vi "Main Tclk.vi"() -> ()   [LabVIEW 2018] (continued)
                n3941 = case shown="True" w3026 {
                  tunnel: w3025 -> [w3034 w3039]
                  tunnel: [w3034 w3039] -> w3024
                  frame False {
                  }
                  frame True {
                    n3942 = Two Button Dialog(message="Are you sure to resume from the last recipe and milling position?") -> (T button?=w3035:bool)  [unwired: 2 in]
                    n3943 = local read "Milling para"() -> (w3036:T35)
                    n3944 = Bundle By Name(cluster=w3036, "Mill start from Last"=w3035) -> (w3037:T35)
                    n3945 = local write "Milling para"(w3037) -> ()
                  }
                }
                n3946 = case shown="2" w3021 {
                  frame 0, Default {
                  }
                  frame 2 {
                    n3947 = local read "Api"() -> (w3033:refnum<k7>)
                    n3948 = local read "FIB Milling Probe"() -> (w3031:string)
                    n3949 = call "SmartSEM Remote API set string.vi"("vValue"=w3031, "lpszParam"="DP_FIB_IMAGE_PROBE", "Api"=w3033) -> ("Api out"=w3030:refnum<k7>)  [unwired: 7 in, 1 out]
                    n3950 = call "SmartSEM Remote API set float.vi"("vValue"="FIB Milling Objective (V)", "lpszParam"="AP_FIB_OBJECTIVE_POTENTIAL", "Api"=w3030) -> ()  [unwired: 7 in, 2 out]
                  }
                }
                n3951 = local write "3D FIB-SEM"(w3024) -> ()
                n3952 = local write "FIB"(w3024) -> ()
                n3953 = case shown="True" w3024 {
                  frame False {
                  }
                  frame True {
                    n3954 = local read "Email Alert Recipients"() -> (w3051:string[])
                    n3955 = local read "Email recipents file"() -> (w3048:path)
                    n3956 = local read "Post #1up"() -> (w3045:tag)
                    n3957 = local read "Post #1down"() -> (w3043:tag)
                    n3958 = local read "Post #2up"() -> (w3044:tag)
                    n3959 = local read "Post #2down"() -> (w3042:tag)
                    n3960 = local write "FIB slice #"(u32 0 ("slice #")) -> ()
                    n3961 = local write "Start FIB HV DataLog"(TRUE ("Start FIB HV DataLog")) -> ()
                    n3962 = local write "Status Tabs"(T11."Status" ("Status Tabs")) -> ()
                    n3963 = Open/Create/Replace File(file path (use dialog)=w3048, operation (0:open)=T49."replace or create") -> (refnum out=w3049:refnum<file>, error out=w3050:errorcluster)  [unwired: 4 in, 1 out]
                    n3964 = call "SEM shutter.vi"("Shutter close"=TRUE, "Shutter AO4"=w3042, "Shutter AO3"=w3044, "Shutter AO2"=w3043, "Shutter AO1"=w3045) -> ()  [unwired: 6 in, 1 out]
                    n3965 = Write to Text File(file (use dialog)=w3049, text=w3051, error in=w3050) -> (refnum out=w3052:refnum<file>, error out=w3053:errorcluster)  [unwired: 1 in, 1 out]
                    n3966 = Close File(refnum=w3052, error in=w3053) -> ()  [unwired: 2 out]
                  }
                }
              }
            }
          }
          event "Pause for reheat": Value Change {
            n3967 = event-data() -> ("NewVal"=w3055:bool)  [unwired: 6 out]
            n3968 = case shown="False" w3055 {
              frame False {
                w3058 = u8 0 ("FI below limit counts")
                n3969 = local read "Machine Type"() -> (w3056:u8)
                n3970 = case shown="1" w3056 {
                  tunnel: [w3064 w3072 w3073] -> w3057
                  frame 0, Default {
                    n3971 = for {
                      N: 10 -> [_]
                      tunnel: [w3069] -> w3066 mode=indexing
                      n3972 = shared-variable ".\\Zeiss Library.lvlib\\Logs"() -> (w3071:sgl[])  [unwired: 1 in, 1 out]
                      n3973 = Wait Until Next ms Multiple(millisecond multiple=u32 10) -> ()  [unwired: 1 out]
                      n3974 = Index Array(array=w3071, index=0) -> (element=w3069:sgl)
                    }
                    n3975 = call-poly <vilib>:"Basic Averaged DC-RMS.vi"("signal in"=w3066) -> ("DC value"=w3065:dbl)  [unwired: 7 in, 3 out]
                    n3976 = To Single Precision Float(number=w3065) -> (single precision float=w3064:sgl)
                  }
                  frame 1 {
                    n3977 = local read "Faraday Cup (nA)"() -> (w3072:sgl)
                  }
                  frame 2 {
                    n3978 = for {
                      N: 10 -> [_]
                      tunnel: [w3078] -> w3075 mode=indexing
                      n3979 = shared-variable ".\\Zeiss Library.lvlib\\Logs"() -> (w3080:sgl[])  [unwired: 1 in, 1 out]
                      n3980 = Wait Until Next ms Multiple(millisecond multiple=u32 10) -> ()  [unwired: 1 out]
                      n3981 = Index Array(array=w3080, index=0) -> (element=w3078:sgl)
                    }
                    n3982 = call-poly <vilib>:"Basic Averaged DC-RMS.vi"("signal in"=w3075) -> ("DC value"=w3074:dbl)  [unwired: 7 in, 3 out]
                    n3983 = To Single Precision Float(number=w3074) -> (single precision float=w3073:sgl)
                  }
                }
                n3984 = local write "FI below limit counts"(w3058) -> ()
                n3985 = local write "FIB CL I out of bound counts"(w3058) -> ()
                n3986 = shared-variable ".\\Zeiss Library.lvlib\\Faraday Cup before mill"(w3057) -> ()  [unwired: 1 in, 1 out]
                n3987 = local write "Faraday Cup before mill"(w3057) -> ()
                n3988 = call <vilib>:"Three Button Dialog.vi"("Allow user to close window? (TRUE)"=FALSE, "Center Button Text (\"No\")"="Manual Re-engage" ("T button name (\"OK\")"), "Left Button Text (\"Yes\")"="Auto Re-engage" ("T button name (\"OK\")"), "message"="Reheat finish and ready to re-engage?") -> ("Which Button?"=w3060:T78)  [unwired: 7 in]
                n3989 = case shown="\"Left Button\"" w3060 {
                  frame "Left Button" {
                    n3990 = stacked-sequence {
                      frame #0 {
                        w3093 = dbl[] [] ("Re-engage Delta X array")
                        w3082 = u8 0 ("Re-engage X shift")
                        w3085 = TRUE ("Auto re-engage")
                        n3991 = local read "X shift from last"() -> (w3087:dbl)
                        n3992 = local read "Y shift from last"() -> (w3091:dbl)
                        n3993 = local read "Reheat from last"() -> (w3088:bool)
                        n3994 = local read "FIB-SEM Angle"() -> (w3096:dbl)
                        n3995 = Get Date/Time In Seconds() -> (seconds since 1Jan1904=w3094:timestamp)
                        "Re-engage time" <- w3094
                        n3996 = local read "Pre-reheat time"() -> (w3097:timestamp)
                        n3997 = Subtract(x=w3094, y=w3097) -> (x-y=w3098:dbl)
                        n3998 = expression code="x/60"(w3098) -> (w3099:dbl)
                        n3999 = expression code="cos(x*pi/180)"(w3096) -> (w3095:dbl)
                        n4000 = Select(t=w3087, s=w3088, f=0.0 ("Re-engage X shift")) -> (s? t:f=w3090:dbl)
                        n4001 = shared-variable ".\\Zeiss Library.lvlib\\FIB PID reset"(w3085) -> ()  [unwired: 1 in, 1 out]
                        n4002 = Natural Logarithm(1:w3099) -> (0:w3101:dbl)
                        n4003 = local write "Re-engage X shift (um)"(w3090) -> ()
                        n4004 = local write "Status message"("Auto re-engaging ..." ("Status message")) -> ()
                        n4005 = Compound Arithmetic op=MULTIPLY(w3095, w3101, 2.5 ("value"), 0.0 ("value")) -> (w3092:dbl)
                        n4006 = Select(t=w3091, s=w3088, f=w3092) -> (s? t:f=w3086:dbl)
                        n4007 = local write "Re-engage Y shift (um)"(w3086) -> ()
                        n4008 = local write "Status Tabs"(T11."Status" ("Status Tabs")) -> ()
                        n4009 = local write "Re-engage counts"(w3082) -> ()
                        n4010 = local write "Recovered counts"(w3082) -> ()
                        n4011 = local write "Last re-engage count"(w3082) -> ()
                        "Auto re-engage" <- w3085
                        "Re-engage Delta X array" <- w3093
                        "Re-engage Delta Y array" <- w3093
                        "Re-engage Y shift array" <- w3093
                        "Re-engage X shift array" <- w3093
                      }
                      frame #1 {
                        w3105 = TRUE ("Reset WD")
                        w3106 = FALSE ("Reheat")
                        n4012 = local write "Config Tabs"(T24."SEM" ("Config Tabs")) -> ()
                        n4013 = local write "Image Tabs"(T37."Detector A" ("Image Tabs")) -> ()
                        n4014 = local write "Pause for reheat"(w3106) -> ()
                        n4015 = local write "Mill Manual Pause"(w3106) -> ()
                        n4016 = local write "Reheat from last"(w3106) -> ()
                        n4017 = property on="Mill Manual Pause" class="Bool (strict)"("DisabledEnum"=T44."Enabled" ("Disabled")) -> ()  [unwired: 2 in, 2 out]
                        n4018 = local write "3D image paused armed"(w3105) -> ()
                        n4019 = local write "SW error warning armed"(w3105) -> ()
                        n4020 = local write "Temperature warning armed"(w3105) -> ()
                        n4021 = local read "Alert Settings"() -> (→"Prior Alert Settings":T36)
                      }
                    }
                  }
                  frame "Center Button", Default {
                    w3111 = TRUE ("Reset WD")
                    w3113 = FALSE ("Reheat")
                    n4022 = local write "3D image paused armed"(w3111) -> ()
                    n4023 = local write "Reset Focus"(w3111) -> ()
                    n4024 = local write "SW error warning armed"(w3111) -> ()
                    n4025 = shared-variable ".\\Zeiss Library.lvlib\\FIB PID reset"(w3111) -> ()  [unwired: 1 in, 1 out]
                    n4026 = local write "Temperature warning armed"(w3111) -> ()
                    n4027 = local write "Config Tabs"(T24."SEM" ("Config Tabs")) -> ()
                    n4028 = local write "Status Tabs"(T11."Status" ("Status Tabs")) -> ()
                    n4029 = local write "Image Tabs"(T37."Detector A" ("Image Tabs")) -> ()
                    n4030 = local write "Pause for reheat"(w3113) -> ()
                    n4031 = local write "Mill Manual Pause"(w3113) -> ()
                    n4032 = local write "Reheat from last"(w3113) -> ()
                    n4033 = property on="Mill Manual Pause" class="Bool (strict)"("DisabledEnum"=T44."Enabled" ("Disabled")) -> ()  [unwired: 2 in, 2 out]
                    n4034 = local write "Status message"("Manual re-engaging ..." ("Status message")) -> ()
                  }
                  frame "Right Button" {
                    n4035 = local write "Pause for reheat"(TRUE ("Reheat request")) -> ()
                  }
                }
              }
              frame True {
                n4036 = local read "Mill Manual Pause"() -> (w3129:bool)
                n4037 = Get Date/Time In Seconds() -> (seconds since 1Jan1904=w3127:timestamp)
                n4038 = local read "3D FIB-SEM Files"() -> (w3119:path)
                n4039 = local read "Re-engage Files"() -> (w3117:path)
                n4040 = local read "Last good FI"() -> (w3126:sgl)
                n4041 = case shown="False" w3129 {
                  frame False {
                    n4042 = stacked-sequence {
                      frame #0 {
                        n4043 = local write "Pause for reheat"(FALSE ("Reheat")) -> ()
                      }
                      frame #1 {
                        n4044 = Two Button Dialog(message="Pause to reheat FIB source?") -> (T button?=w3131:bool)  [unwired: 2 in]
                        n4045 = local write "Pause for reheat"(w3131) -> ()
                        n4046 = case shown="True" w3131 {
                          frame False {
                          }
                          frame True {
                            n4047 = local write "Reheat completed"(FALSE ("Reheat completed")) -> ()
                            n4048 = local write "Status message"("Pausing for FIB reheat ..." ("Status message")) -> ()
                            n4049 = property on="Pause for reheat" class="Bool (strict)"("DisabledEnum"=T44."Disabled and Grayed Out" ("Disabled")) -> ()  [unwired: 2 in, 2 out]
                          }
                        }
                      }
                    }
                  }
                  frame True {
                    n4050 = property on="Mill Manual Pause" class="Bool (strict)"("DisabledEnum"=T44."Disabled and Grayed Out" ("Disabled")) -> ()  [unwired: 2 in, 2 out]
                  }
                }
                n4051 = local read "SEM Scan Parameters"() -> (w3128:T26)
                n4052 = Build Path(base path=w3119, name or relative path="LG low res.png") -> (appended path=w3120:path)
                n4053 = Build Path(base path=w3117, name or relative path="pre.png") -> (appended path=w3121:path)
                n4054 = local write "Pre-reheat time"(w3127) -> ()
                n4055 = Copy(9:TRUE ("overwrite (F)"), 10:w3121, 11:w3120) -> ()  [unwired: 2 in, 3 out]
                n4056 = local write "Pre-reheat FI"(w3126) -> ()
                n4057 = Unbundle By Name(w3128) -> ("X center (um)"=w3125:sgl, "Y center (um)"=w3124:sgl, "Y stig"=w3123:sgl[][])
                n4058 = local write "Pre-reheat X center (um)"(w3125) -> ()
                n4059 = local write "Pre-reheat Y center (um)"(w3124) -> ()
                n4060 = local write "Pre-reheat Y stig"(w3123) -> ()
              }
            }
          }
          event "FIB Imaging": Mouse Down {
            n4061 = event-data() -> ("PlatMods"=w3138:T77)  [unwired: 7 out]
            n4062 = Unbundle By Name(w3138) -> ("Shift"=→"FIB single scan":bool)
          }
          event "FIB Imaging": Value Change {
            n4063 = event-data() -> ("NewVal"=w3139:bool)  [unwired: 5 out]
            n4064 = case shown="True" w3139 {
              selector: w3139 -> [w3140 _]
              frame False {
                n4065 = local write "Unfreeze"(w3140) -> ()
                n4066 = stacked-sequence {
                  frame #0 {
                    n4067 = shared-variable "My Computer\\Zeiss Library.lvlib\\Realtime Imaging stop"(TRUE ("Realtime Imaging stop")) -> ()  [unwired: 1 in, 1 out]
                  }
                  frame #1 {
                    n4068 = disable-structure shown="Disabled" {
                      frame Disabled {
                        n4069 = local read "Machine Type"() -> (w3142:u8)
                        n4070 = case shown="1" w3142 {
                          frame 0, Default {
                          }
                          frame 1 {
                            n4071 = stacked-sequence {
                              frame #0 {
                                n4072 = Wait (ms)(milliseconds to wait=u32 1000) -> ()  [unwired: 1 out]
                              }
                              frame #1 {
                                w3144 = TRUE ("Initialization")
                                n4073 = local read "COM port"() -> (w3150:refnum<visa-resource-name>)
                                n4074 = call "FIB mode.vi"("Initialization"=w3144, "FIB mode"=T10."SEM", "COM port in"=w3150) -> ("COM port out"=w3149:refnum<visa-resource-name>)  [unwired: 7 in, 1 out]
                                n4075 = call "Remcon32 command.vi"("SEM command"="edx 0", "COM port in"=w3149) -> ("COM port out"=w3148:refnum<visa-resource-name>)  [unwired: 6 in, 3 out]
                                n4076 = call "Remcon32 command.vi"("Close session"=w3144, "SEM command"="frez", "COM port in"=w3148) -> ()  [unwired: 5 in, 4 out]
                              }
                            }
                          }
                          frame 2 {
                          }
                        }
                      }
                      frame Enabled {
                      }
                    }
                  }
                  frame #2 {
                    w3152 = T44."Enabled" ("Disabled")
                    n4077 = local write "Status message"("standby" ("Status message")) -> ()
                    n4078 = property on="Pre image" class="Bool (strict)"("DisabledEnum"=w3152) -> ()  [unwired: 2 in, 2 out]
                    n4079 = property on="Post image" class="Bool (strict)"("DisabledEnum"=w3152) -> ()  [unwired: 2 in, 2 out]
                    n4080 = local read "FIB"() -> (w3153:bool)
                    n4081 = property on="Mill Manual Pause" class="Bool (strict)"("DisabledEnum"=w3152) -> ()  [unwired: 2 in, 2 out]
                    n4082 = case shown="False" w3153 {
                      tunnel: w3152 -> [w3154 _]
                      frame False {
                        n4083 = property on="Mill" class="Bool (strict)"("DisabledEnum"=w3154) -> ()  [unwired: 2 in, 2 out]
                      }
                      frame True {
                      }
                    }
                  }
                }
              }
              frame True {
                n4084 = local read "Machine Type"() -> (w3156:u8)
                n4085 = case shown="2" w3156 {
                  tunnel: [TRUE ("true") w3168] -> w3155
                  frame 0, Default {
                  }
                  frame 2 {
                    n4086 = local read "Api"() -> (w3166:refnum<k7>)
                    n4087 = Two Button Dialog(message="Verify if FIB probe is at 50 pA") -> (T button?=w3168:bool)  [unwired: 2 in]
                    n4088 = call "SmartSEM Remote API set string.vi"("vValue"="FIB Imaging Probe", "lpszParam"="DP_FIB_IMAGE_PROBE", "Api"=w3166) -> ()  [unwired: 7 in, 2 out]
                  }
                }
                "Unfreeze" <- w3155
                n4089 = case shown="True" w3155 {
                  frame False {
                  }
                  frame True {
                    n4090 = stacked-sequence {
                      frame #0 {
                        n4091 = local read "Spot"() -> (w3157:bool)
                        n4092 = case shown="True" w3157 {
                          frame False {
                          }
                          frame True {
                            n4093 = local write "Spot"(FALSE ("Spot")) -> ()
                            n4094 = Wait (ms)(milliseconds to wait=u32 200) -> ()  [unwired: 1 out]
                          }
                        }
                      }
                      frame #1 {
                        w3162 = T44."Disabled and Grayed Out" ("Disabled")
                        n4095 = local write "Status message"("FIB Imaging" ("Status message")) -> ()
                        n4096 = local write "Image Tabs"(T37."FIB" ("Image Tabs")) -> ()
                        n4097 = local write "Status Tabs"(T11."FIB" ("Status Tabs")) -> ()
                        n4098 = property on="Pre image" class="Bool (strict)"("DisabledEnum"=w3162) -> ()  [unwired: 2 in, 2 out]
                        n4099 = property on="Post image" class="Bool (strict)"("DisabledEnum"=w3162) -> ()  [unwired: 2 in, 2 out]
                        n4100 = property on="Mill" class="Bool (strict)"("DisabledEnum"=w3162) -> ()  [unwired: 2 in, 2 out]
                        n4101 = property on="Mill Manual Pause" class="Bool (strict)"("DisabledEnum"=w3162) -> ()  [unwired: 2 in, 2 out]
                      }
                    }
                  }
                }
                n4102 = local write "FIB Imaging"(w3155) -> ()
              }
            }
          }
          event "Update": Value Change {
            n4103 = event-data() -> ("NewVal"=w3170:bool)  [unwired: 5 out]
            n4104 = case shown="True" w3170 {
              frame False {
              }
              frame True {
                n4105 = stacked-sequence {
                  frame #0 {
                    n4106 = local write "Unfreeze"(FALSE ("FIB beam blank")) -> ()
                    n4107 = shared-variable "My Computer\\Zeiss Library.lvlib\\Realtime Imaging stop"(TRUE ("Realtime Imaging stop")) -> ()  [unwired: 1 in, 1 out]
                  }
                  frame #1 {
                    n4108 = Wait (ms)(milliseconds to wait=u32 1000) -> ()  [unwired: 1 out]
                  }
                  frame #2 {
                    n4109 = local write "Unfreeze"(TRUE ("Realtime Imaging stop")) -> ()
                  }
                }
              }
            }
          }
          event "Reset": Value Change {
            n4110 = event-data() -> ("NewVal"=w3175:bool)  [unwired: 5 out]
            n4111 = case shown="True" w3175 {
              frame False {
              }
              frame True {
                n4112 = stacked-sequence {
                  frame #0 {
                    n4113 = local read "SEM HW Config"() -> (w3186:T9)
                    n4114 = local read "FIB HW Config"() -> (w3178:T23)
                    n4115 = Unbundle By Name(w3186) -> ("SEM X coil"=w3185:refnum<k15>)
                    n4116 = Unbundle By Name(w3178) -> ("FIB X coil"=w3177:tag)
                    n4117 = Type Cast(x=w3185) -> (*(type *) &x=w3184:string)  [unwired: 1 in]
                    n4118 = Type Cast(x=w3177) -> (*(type *) &x=w3179:string)  [unwired: 1 in]
                    n4119 = Match Pattern(string=w3184, regular expression="/") -> (before substring=w3182:string)  [unwired: 1 in, 3 out]
                    n4120 = Match Pattern(string=w3179, regular expression="/") -> (before substring=w3181:string)  [unwired: 1 in, 3 out]
                    n4121 = call <vilib>:"DAQmx Reset Device.vi"("device in"=w3182) -> ()  [unwired: 14 in, 1 out]
                    n4122 = call <vilib>:"DAQmx Reset Device.vi"("device in"=w3181) -> ()  [unwired: 14 in, 1 out]
                    n4123 = shared-variable ".\\Zeiss Library.lvlib\\Force tclk init"(TRUE ("Force tclk init")) -> ()  [unwired: 1 in, 1 out]
                  }
                  frame #1 {
                    n4124 = local read "FIB HW Config"() -> (w3194:T23)
                    n4125 = Unbundle By Name(w3194) -> ("Beam blank"=w3195:tag)
                    n4126 = local read "Api"() -> (w3187:refnum<k7>)
                    n4127 = call "FIB beam blank.vi"("Api"=w3187, "Beam blanked"=TRUE ("Ext on"), "lines"=w3195) -> ()  [unwired: 2 in, 1 out]
                    n4128 = local read "Post #1up"() -> (w3191:tag)
                    n4129 = local read "Post #1down"() -> (w3190:tag)
                    n4130 = local read "Post #2up"() -> (w3189:tag)
                    n4131 = local read "Post #2down"() -> (w3188:tag)
                    n4132 = call "SEM shutter.vi"("Shutter close"=FALSE, "Shutter AO4"=w3188, "Shutter AO3"=w3189, "Shutter AO2"=w3190, "Shutter AO1"=w3191) -> ()  [unwired: 6 in, 1 out]
                  }
                  frame #2 {
                    n4133 = local read "SEM HW Config"() -> (w3200:T9)
                    n4134 = Unbundle By Name(w3200) -> ("Detector FIB-NI auto switch"=w3201:tag)
                    n4135 = call-poly <vilib>:"DAQmx Create Virtual Channel.vi"("lines"=w3201) -> ("task out"=w3198:refnum<k21>, "error out"=w3199:errorcluster)  [unwired: 4 in, 9 out]
                    n4136 = call-poly <vilib>:"DAQmx Write.vi"("task/channels in"=w3198, "data"=FALSE, "error in"=w3199) -> ("task out"=w3196:refnum<k21>, "error out"=w3197:errorcluster)  [unwired: 1 in, 10 out]
                    n4137 = call <vilib>:"DAQmx Clear Task.vi"("task in"=w3196, "error in"=w3197) -> ()  [unwired: 14 out]
                  }
                  frame #3 {
                    n4138 = local read "FIB HW Config"() -> (w3205:T23)
                    n4139 = Unbundle By Name(w3205) -> ("FIB Ext Scan"=w3204:tag)
                    n4140 = call "FIB ext scan.vi"("Ext on"=FALSE, "FIB Ext Scan"=w3204) -> ()  [unwired: 9 in, 1 out]
                  }
                  frame #4 {
                    n4141 = local read "Machine Type"() -> (w3206:u8)
                    n4142 = case shown="2" w3206 {
                      frame 0, Default {
                      }
                      frame 1 {
                        w3207 = TRUE ("Initialization")
                        n4143 = local read "COM port"() -> (w3213:refnum<visa-resource-name>)
                        n4144 = call "FIB mode.vi"("Initialization"=w3207, "FIB mode"=T10."SEM", "COM port in"=w3213) -> ("COM port out"=w3212:refnum<visa-resource-name>)  [unwired: 7 in, 1 out]
                        n4145 = call "Remcon32 command.vi"("SEM command"="edx 0", "COM port in"=w3212) -> ("COM port out"=w3211:refnum<visa-resource-name>)  [unwired: 6 in, 3 out]
                        n4146 = call "Remcon32 command.vi"("Close session"=w3207, "SEM command"="frez", "COM port in"=w3211) -> ()  [unwired: 5 in, 4 out]
                      }
                      frame 2 {
                        n4147 = local read "Api"() -> (w3214:refnum<k7>)
                        n4148 = call "SmartSEM Remote API set float.vi"("vValue"=sgl 0.0, "lpszParam"="DP_PANEL_DISABLE", "Api"=w3214) -> ("Api out"=w3215:refnum<k7>)  [unwired: 7 in, 1 out]
                        n4149 = call "SmartSEM Remote API set float.vi"("vValue"=sgl 0.0, "lpszParam"="DP_JOYSTICK_DISABLE", "Api"=w3215) -> ()  [unwired: 7 in, 2 out]
                      }
                    }
                  }
                  frame #5 {
                    n4150 = local write "Reset"(FALSE ("Reset")) -> ()
                  }
                }
              }
            }
          }
          event "Off": Value Change {
            n4151 = event-data() -> ("NewVal"=w3221:bool)  [unwired: 6 out]
            n4152 = case shown="False" w3221 {
              tunnel: [FALSE ("T button?") w3224] -> w3222
              frame False {
              }
              frame True {
                n4153 = local read "FIB"() -> (w3225:bool)
                n4154 = Two Button Dialog(message="Stop Program?") -> (T button?=w3226:bool)  [unwired: 2 in]
                n4155 = case shown="True" w3225 {
                  tunnel: w3226 -> [w3228 w3229]
                  tunnel: [w3228 w3229] -> w3224
                  frame False {
                    n4156 = shared-variable "My Computer\\Zeiss Library.lvlib\\Stop"(w3228) -> ()  [unwired: 1 in, 1 out]
                    n4157 = shared-variable "My Computer\\Zeiss Library.lvlib\\Milling Stop"(w3228) -> ()  [unwired: 1 in, 1 out]
                    n4158 = shared-variable "My Computer\\Zeiss Library.lvlib\\Realtime Imaging stop"(w3228) -> ()  [unwired: 1 in, 1 out]
                    n4159 = local write "Stop"(w3228) -> ()
                    n4160 = local write "Off"(w3228) -> ()
                  }
                  frame True {
                    n4161 = shared-variable "My Computer\\Zeiss Library.lvlib\\Stop"(w3229) -> ()  [unwired: 1 in, 1 out]
                    n4162 = shared-variable "My Computer\\Zeiss Library.lvlib\\Milling Stop"(w3229) -> ()  [unwired: 1 in, 1 out]
                    n4163 = shared-variable "My Computer\\Zeiss Library.lvlib\\Realtime Imaging stop"(w3229) -> ()  [unwired: 1 in, 1 out]
                    n4164 = local write "Stop"(w3229) -> ()
                    n4165 = local write "Off"(w3229) -> ()
                  }
                }
              }
            }
          }
          event "SEM Scan Parameters": Value Change {
            w3231 = sgl[] [] ("Delta X array for stop limit")
            n4166 = event-data() -> ()  [unwired: 6 out]
            n4167 = local write "SW error warning armed"(FALSE ("SW error warning armed")) -> ()
            n4168 = local write "Cycle time array"(u32[] [] ("Cycle time array")) -> ()
            n4169 = local write "Cycle time est offset array"(i16[] [] ("Cycle time array")) -> ()
            n4170 = local write "Continued fine milling frames"(0 ("Continued fine milling frames")) -> ()
            n4171 = local write "FI array for stop limit"(w3231) -> ()
            n4172 = local write "Delta X array for stop limit"(w3231) -> ()
            n4173 = local write "Delta Y array for stop limit"(w3231) -> ()
          }
          event "SEM Scan Parameters.X tiles": Value Change {
            n4174 = event-data() -> ("OldVal"=w3239:u8, "NewVal"=w3238:u8)  [unwired: 5 out]
            n4175 = In Range and Coerce(upper limit=u8 255, x=w3238, lower limit=u8 1) -> (coerced(x)=w3237:u8)  [unwired: 1 out]
            n4176 = call <vilib>:"Three Button Dialog.vi"("Center Button Text (\"No\")"="Manual" ("Center Button Text (\"No\")"), "Left Button Text (\"Yes\")"="Auto" ("message"), "message"="Modify WD, Stig, and Aperture Align?") -> ("Which Button?"=w3242:T78)  [unwired: 8 in]
            n4177 = case shown="\"Left Button\"" w3242 {
              tunnel: w3237 -> [w3244 w3274 _]
              tunnel: w3239 -> [_ _ w3350]
              frame "Left Button" {
                n4178 = local read "SEM Scan Parameters"() -> (w3260:T26)
                n4179 = Unbundle By Name(w3260) -> ("X stig"=w3266:sgl[][], "Y stig"=w3265:sgl[][], "X aln"=w3264:sgl[][], "Y aln"=w3263:sgl[][], "WD (mm)"=w3262:sgl[][], "dY (um)"=w3251:sgl[], "Y tiles"=w3245:u8)
                n4180 = Build Array(w3266, w3265, w3264, w3263, w3262) -> (w3261:sgl[][][])
                n4181 = for {
                  tunnel: w3261 -> [w3269] mode=indexing
                  tunnel: w3244 -> [w3268]
                  tunnel: [w3267] -> w3258 mode=indexing
                  workers-P: _ -> [_]
                  n4182 = for {
                    tunnel: w3269 -> [w3273] mode=indexing
                    tunnel: w3268 -> [w3271]
                    tunnel: [w3270] -> w3267 mode=indexing
                    workers-P: _ -> [_]
                    n4183 = call-poly <vilib>:"Mean.vi"("X"=w3273) -> ("mean"=w3272:dbl)  [unwired: 1 out]
                    n4184 = Initialize Array(w3272, w3271) -> (w3270:dbl[])
                  }
                }
                n4185 = call-poly <vilib>:"Mean.vi"("X"=w3251) -> ("mean"=w3252:dbl)  [unwired: 1 out]
                n4186 = Initialize Array(w3252, w3244) -> (w3250:dbl[])
                n4187 = Initialize Array(u8 1 ("element"), w3245, w3244) -> (w3246:u8[][])
                n4188 = local read "Focus Index Options"() -> (w3248:T28)
                n4189 = Index Array(array=w3258) -> (element #1=w3257:dbl[][], element #2=w3256:dbl[][], element #3=w3255:dbl[][], element #4=w3254:dbl[][], element #5=w3253:dbl[][])  [unwired: 15 in]
                n4190 = Bundle By Name(cluster=w3248, "X Grids"=w3246, "Y Grids"=w3246, "Primary X index"=w3246, "Primary Y index"=w3246) -> (w3247:T28)
                n4191 = Bundle By Name(cluster=w3260, "X stig"=w3257, "Y stig"=w3256, "X aln"=w3255, "Y aln"=w3254, "WD (mm)"=w3253, "dY (um)"=w3250, "X tiles"=w3244) -> (w3259:T26)
                n4192 = local write "SEM Scan Parameters"(w3259) -> ()
                n4193 = local write "Focus Index Options"(w3247) -> ()
              }
              frame "Center Button" {
                n4194 = stacked-sequence {
                  tunnel: w3274 -> [w3275 w3292 w3303 w3315 w3327 w3340]
                  frame #0 {
                    n4195 = local read "SEM Scan Parameters"() -> (w3288:T26)
                    n4196 = Unbundle By Name(w3288) -> ("WD (mm)"=w3290:sgl[][], "Y tiles"=w3276:u8)
                    n4197 = call "2D array edit.vi"("Data Entry Limits:Increment"=0.001, "Display Format:Precision"=u8 4, "Rows"=w3276, "Columns"=w3275, "Caption.Text"="WD (mm)", "Input array"=w3290) -> ("Output array"=w3286:sgl[][])  [unwired: 5 in]
                    n4198 = Array Size(array=w3286) -> (size(s)=w3285:i32[])
                    n4199 = Initialize Array(u8 1 ("element"), w3276, w3275) -> (w3277:u8[][])
                    n4200 = local read "Focus Index Options"() -> (w3279:T28)
                    n4201 = Index Array(array=w3285) -> (element #1=w3284:i32, element #2=w3283:i32)  [unwired: 2 in]
                    n4202 = Bundle By Name(cluster=w3279, "X Grids"=w3277, "Y Grids"=w3277, "Primary X index"=w3277, "Primary Y index"=w3277) -> (w3278:T28)
                    n4203 = Bundle By Name(cluster=w3288, "WD (mm)"=w3286, "X tiles"=w3283, "Y tiles"=w3284) -> (w3287:T26)
                    n4204 = local write "SEM Scan Parameters"(w3287) -> ()
                    n4205 = local write "Focus Index Options"(w3278) -> ()
                  }
                  frame #1 {
                    n4206 = local read "SEM Scan Parameters"() -> (w3300:T26)
                    n4207 = Unbundle By Name(w3300) -> ("X stig"=w3302:sgl[][], "Y tiles"=w3291:u8)
                    n4208 = call "2D array edit.vi"("Data Entry Limits:Increment"=0.1, "Display Format:Precision"=u8 2, "Rows"=w3291, "Columns"=w3292, "Caption.Text"="X stig (%)", "Input array"=w3302) -> ("Output array"=w3297:sgl[][])  [unwired: 5 in]
                    n4209 = Array Size(array=w3297) -> (size(s)=w3298:i32[])
                    n4210 = Index Array(array=w3298) -> (element #1=w3296:i32, element #2=w3295:i32)  [unwired: 2 in]
                    n4211 = Bundle By Name(cluster=w3300, "X stig"=w3297, "X tiles"=w3295, "Y tiles"=w3296) -> (w3299:T26)
                    n4212 = local write "SEM Scan Parameters"(w3299) -> ()
                  }
                  frame #2 {
                    n4213 = local read "SEM Scan Parameters"() -> (w3312:T26)
                    n4214 = Unbundle By Name(w3312) -> ("Y stig"=w3314:sgl[][], "Y tiles"=w3310:u8)
                    n4215 = call "2D array edit.vi"("Data Entry Limits:Increment"=0.1, "Display Format:Precision"=u8 2, "Rows"=w3310, "Columns"=w3303, "Caption.Text"="Y stig (%)", "Input array"=w3314) -> ("Output array"=w3308:sgl[][])  [unwired: 5 in]
                    n4216 = Array Size(array=w3308) -> (size(s)=w3309:i32[])
                    n4217 = Index Array(array=w3309) -> (element #1=w3307:i32, element #2=w3306:i32)  [unwired: 2 in]
                    n4218 = Bundle By Name(cluster=w3312, "Y stig"=w3308, "X tiles"=w3306, "Y tiles"=w3307) -> (w3311:T26)
                    n4219 = local write "SEM Scan Parameters"(w3311) -> ()
                  }
                  frame #3 {
                    n4220 = local read "SEM Scan Parameters"() -> (w3324:T26)
                    n4221 = Unbundle By Name(w3324) -> ("X aln"=w3326:sgl[][], "Y tiles"=w3322:u8)
                    n4222 = call "2D array edit.vi"("Data Entry Limits:Increment"=0.1, "Display Format:Precision"=u8 2, "Rows"=w3322, "Columns"=w3315, "Caption.Text"="X aln (%)", "Input array"=w3326) -> ("Output array"=w3320:sgl[][])  [unwired: 5 in]
                    n4223 = Array Size(array=w3320) -> (size(s)=w3321:i32[])
                    n4224 = Index Array(array=w3321) -> (element #1=w3319:i32, element #2=w3318:i32)  [unwired: 2 in]
                    n4225 = Bundle By Name(cluster=w3324, "X aln"=w3320, "X tiles"=w3318, "Y tiles"=w3319) -> (w3323:T26)
                    n4226 = local write "SEM Scan Parameters"(w3323) -> ()
                  }
                  frame #4 {
                    n4227 = local read "SEM Scan Parameters"() -> (w3336:T26)
                    n4228 = Unbundle By Name(w3336) -> ("Y aln"=w3338:sgl[][], "Y tiles"=w3334:u8)
                    n4229 = call "2D array edit.vi"("Data Entry Limits:Increment"=0.1, "Display Format:Precision"=u8 2, "Rows"=w3334, "Columns"=w3327, "Caption.Text"="Y aln (%)", "Input array"=w3338) -> ("Output array"=w3332:sgl[][])  [unwired: 5 in]
                    n4230 = Array Size(array=w3332) -> (size(s)=w3333:i32[])
                    n4231 = Index Array(array=w3333) -> (element #1=w3331:i32, element #2=w3330:i32)  [unwired: 2 in]
                    n4232 = Bundle By Name(cluster=w3336, "Y aln"=w3332, "X tiles"=w3330, "Y tiles"=w3331) -> (w3335:T26)
                    n4233 = local write "SEM Scan Parameters"(w3335) -> ()
                  }
                  frame #5 {
                    w3343 = u8 1 ("Rows")
                    n4234 = local read "SEM Scan Parameters"() -> (w3348:T26)
                    n4235 = Unbundle By Name(w3348) -> ("dY (um)"=w3344:sgl[])
                    n4236 = Reshape Array(w3344, w3343, w3340) -> (w3342:sgl[][])
                    n4237 = call "2D array edit.vi"("Data Entry Limits:Increment"=0.1, "Display Format:Precision"=u8 2, "Rows"=w3343, "Columns"=w3340, "Caption.Text"="dY (um)", "Input array"=w3342) -> ("Output array"=w3341:sgl[][])  [unwired: 5 in]
                    n4238 = Reshape Array(w3341, w3340) -> (w3339:sgl[])
                    n4239 = Bundle By Name(cluster=w3348, "dY (um)"=w3339, "X tiles"=w3340) -> (w3347:T26)
                    n4240 = local write "SEM Scan Parameters"(w3347) -> ()
                  }
                }
              }
              frame "Right Button", Default {
                n4241 = local read "SEM Scan Parameters"() -> (w3351:T26)
                n4242 = Bundle By Name(cluster=w3351, "X tiles"=w3350) -> (w3352:T26)
                n4243 = local write "SEM Scan Parameters"(w3352) -> ()
              }
            }
          }
          event "SEM Scan Parameters.Y tiles": Value Change {
            n4244 = event-data() -> ("OldVal"=w3357:u8, "NewVal"=w3356:u8)  [unwired: 5 out]
            n4245 = In Range and Coerce(upper limit=u8 255, x=w3356, lower limit=u8 1) -> (coerced(x)=w3355:u8)  [unwired: 1 out]
            n4246 = call <vilib>:"Three Button Dialog.vi"("Center Button Text (\"No\")"="Manual" ("Center Button Text (\"No\")"), "Left Button Text (\"Yes\")"="Auto" ("message"), "message"="Modify WD, Stig, and Aperture Align?") -> ("Which Button?"=w3358:T78)  [unwired: 8 in]
            n4247 = case shown="\"Left Button\"" w3358 {
              tunnel: w3355 -> [w3363 w3394 _]
              tunnel: w3357 -> [_ _ w3470]
              frame "Left Button" {
                n4248 = local read "SEM Scan Parameters"() -> (w3378:T26)
                n4249 = Unbundle By Name(w3378) -> ("X stig"=w3384:sgl[][], "Y stig"=w3383:sgl[][], "X aln"=w3382:sgl[][], "Y aln"=w3381:sgl[][], "WD (mm)"=w3380:sgl[][], "dX (um)"=w3369:sgl[], "X tiles"=w3362:u8)
                n4250 = Build Array(w3384, w3383, w3382, w3381, w3380) -> (w3379:sgl[][][])
                n4251 = for {
                  tunnel: w3379 -> [w3388] mode=indexing
                  tunnel: w3363 -> [w3389]
                  tunnel: [w3385] -> w3376 mode=indexing
                  workers-P: _ -> [_]
                  n4252 = Transpose 2D Array(2D array=w3388) -> (transposed array=w3387:sgl[][])
                  n4253 = for {
                    tunnel: w3389 -> [w3392]
                    tunnel: [w3391] -> w3386 mode=indexing
                    workers-P: _ -> [_]
                    tunnel: w3387 -> [w3390] mode=indexing
                    n4254 = call-poly <vilib>:"Mean.vi"("X"=w3390) -> ("mean"=w3393:dbl)  [unwired: 1 out]
                    n4255 = Initialize Array(w3393, w3392) -> (w3391:dbl[])
                  }
                  n4256 = Transpose 2D Array(2D array=w3386) -> (transposed array=w3385:dbl[][])
                }
                n4257 = call-poly <vilib>:"Mean.vi"("X"=w3369) -> ("mean"=w3370:dbl)  [unwired: 1 out]
                n4258 = Initialize Array(w3370, w3363) -> (w3368:dbl[])
                n4259 = Index Array(array=w3376) -> (element #1=w3375:dbl[][], element #2=w3374:dbl[][], element #3=w3373:dbl[][], element #4=w3372:dbl[][], element #5=w3371:dbl[][])  [unwired: 15 in]
                n4260 = Initialize Array(u8 1 ("element"), w3363, w3362) -> (w3364:u8[][])
                n4261 = local read "Focus Index Options"() -> (w3366:T28)
                n4262 = Bundle By Name(cluster=w3366, "X Grids"=w3364, "Y Grids"=w3364, "Primary X index"=w3364, "Primary Y index"=w3364) -> (w3365:T28)
                n4263 = Bundle By Name(cluster=w3378, "X stig"=w3375, "Y stig"=w3374, "X aln"=w3373, "Y aln"=w3372, "WD (mm)"=w3371, "dX (um)"=w3368, "Y tiles"=w3363) -> (w3377:T26)
                n4264 = local write "SEM Scan Parameters"(w3377) -> ()
                n4265 = local write "Focus Index Options"(w3365) -> ()
              }
              frame "Center Button" {
                n4266 = stacked-sequence {
                  tunnel: w3394 -> [w3395 w3411 w3423 w3435 w3447 w3460]
                  frame #0 {
                    n4267 = local read "SEM Scan Parameters"() -> (w3408:T26)
                    n4268 = Unbundle By Name(w3408) -> ("WD (mm)"=w3410:sgl[][], "X tiles"=w3396:u8)
                    n4269 = call "2D array edit.vi"("Data Entry Limits:Increment"=0.001, "Display Format:Precision"=u8 4, "Rows"=w3395, "Columns"=w3396, "Caption.Text"="WD (mm)", "Input array"=w3410) -> ("Output array"=w3406:sgl[][])  [unwired: 5 in]
                    n4270 = Array Size(array=w3406) -> (size(s)=w3405:i32[])
                    n4271 = Initialize Array(u8 1 ("element"), w3395, w3396) -> (w3397:u8[][])
                    n4272 = local read "Focus Index Options"() -> (w3399:T28)
                    n4273 = Index Array(array=w3405) -> (element #1=w3404:i32, element #2=w3403:i32)  [unwired: 2 in]
                    n4274 = Bundle By Name(cluster=w3399, "X Grids"=w3397, "Y Grids"=w3397, "Primary X index"=w3397, "Primary Y index"=w3397) -> (w3398:T28)
                    n4275 = Bundle By Name(cluster=w3408, "WD (mm)"=w3406, "X tiles"=w3403, "Y tiles"=w3404) -> (w3407:T26)
                    n4276 = local write "SEM Scan Parameters"(w3407) -> ()
                    n4277 = local write "Focus Index Options"(w3398) -> ()
                  }
                  frame #1 {
                    n4278 = local read "SEM Scan Parameters"() -> (w3420:T26)
                    n4279 = Unbundle By Name(w3420) -> ("X stig"=w3422:sgl[][], "X tiles"=w3412:u8)
                    n4280 = call "2D array edit.vi"("Data Entry Limits:Increment"=0.1, "Display Format:Precision"=u8 2, "Rows"=w3411, "Columns"=w3412, "Caption.Text"="X stig (%)", "Input array"=w3422) -> ("Output array"=w3417:sgl[][])  [unwired: 5 in]
                    n4281 = Array Size(array=w3417) -> (size(s)=w3418:i32[])
                    n4282 = Index Array(array=w3418) -> (element #1=w3416:i32, element #2=w3415:i32)  [unwired: 2 in]
                    n4283 = Bundle By Name(cluster=w3420, "X stig"=w3417, "X tiles"=w3415, "Y tiles"=w3416) -> (w3419:T26)
                    n4284 = local write "SEM Scan Parameters"(w3419) -> ()
                  }
                  frame #2 {
                    n4285 = local read "SEM Scan Parameters"() -> (w3432:T26)
                    n4286 = Unbundle By Name(w3432) -> ("Y stig"=w3434:sgl[][], "X tiles"=w3424:u8)
                    n4287 = call "2D array edit.vi"("Data Entry Limits:Increment"=0.1, "Display Format:Precision"=u8 2, "Rows"=w3423, "Columns"=w3424, "Caption.Text"="Y stig (%)", "Input array"=w3434) -> ("Output array"=w3429:sgl[][])  [unwired: 5 in]
                    n4288 = Array Size(array=w3429) -> (size(s)=w3430:i32[])
                    n4289 = Index Array(array=w3430) -> (element #1=w3428:i32, element #2=w3427:i32)  [unwired: 2 in]
                    n4290 = Bundle By Name(cluster=w3432, "Y stig"=w3429, "X tiles"=w3427, "Y tiles"=w3428) -> (w3431:T26)
                    n4291 = local write "SEM Scan Parameters"(w3431) -> ()
                  }
                  frame #3 {
                    n4292 = local read "SEM Scan Parameters"() -> (w3444:T26)
                    n4293 = Unbundle By Name(w3444) -> ("X aln"=w3446:sgl[][], "X tiles"=w3436:u8)
                    n4294 = call "2D array edit.vi"("Data Entry Limits:Increment"=0.1, "Display Format:Precision"=u8 2, "Rows"=w3435, "Columns"=w3436, "Caption.Text"="X aln (%)", "Input array"=w3446) -> ("Output array"=w3441:sgl[][])  [unwired: 5 in]
                    n4295 = Array Size(array=w3441) -> (size(s)=w3442:i32[])
                    n4296 = Index Array(array=w3442) -> (element #1=w3440:i32, element #2=w3439:i32)  [unwired: 2 in]
                    n4297 = Bundle By Name(cluster=w3444, "X aln"=w3441, "X tiles"=w3439, "Y tiles"=w3440) -> (w3443:T26)
                    n4298 = local write "SEM Scan Parameters"(w3443) -> ()
                  }
                  frame #4 {
                    n4299 = local read "SEM Scan Parameters"() -> (w3456:T26)
                    n4300 = Unbundle By Name(w3456) -> ("Y aln"=w3458:sgl[][], "X tiles"=w3448:u8)
                    n4301 = call "2D array edit.vi"("Data Entry Limits:Increment"=0.1, "Display Format:Precision"=u8 2, "Rows"=w3447, "Columns"=w3448, "Caption.Text"="Y aln (%)", "Input array"=w3458) -> ("Output array"=w3453:sgl[][])  [unwired: 5 in]
                    n4302 = Array Size(array=w3453) -> (size(s)=w3454:i32[])
                    n4303 = Index Array(array=w3454) -> (element #1=w3452:i32, element #2=w3451:i32)  [unwired: 2 in]
                    n4304 = Bundle By Name(cluster=w3456, "Y aln"=w3453, "X tiles"=w3451, "Y tiles"=w3452) -> (w3455:T26)
                    n4305 = local write "SEM Scan Parameters"(w3455) -> ()
                  }
                  frame #5 {
                    w3459 = u8 1 ("Rows")
                    n4306 = local read "SEM Scan Parameters"() -> (w3468:T26)
                    n4307 = Unbundle By Name(w3468) -> ("dX (um)"=w3464:sgl[])
                    n4308 = Reshape Array(w3464, w3460, w3459) -> (w3463:sgl[][])
                    n4309 = call "2D array edit.vi"("Data Entry Limits:Increment"=0.1, "Display Format:Precision"=u8 2, "Rows"=w3460, "Columns"=w3459, "Caption.Text"="dX (um)", "Input array"=w3463) -> ("Output array"=w3462:sgl[][])  [unwired: 5 in]
                    n4310 = Reshape Array(w3462, w3460) -> (w3461:sgl[])
                    n4311 = Bundle By Name(cluster=w3468, "dX (um)"=w3461, "Y tiles"=w3460) -> (w3467:T26)
                    n4312 = local write "SEM Scan Parameters"(w3467) -> ()
                  }
                }
              }
              frame "Right Button", Default {
                n4313 = local read "SEM Scan Parameters"() -> (w3471:T26)
                n4314 = Bundle By Name(cluster=w3471, "Y tiles"=w3470) -> (w3472:T26)
                n4315 = local write "SEM Scan Parameters"(w3472) -> ()
              }
            }
          }
          event "SEM Scan Parameters.WD (mm)": Mouse Down; "SEM Scan Parameters.WD (mm)": Value Change {
            n4316 = event-data() -> ()  [unwired: 5 out]
            n4317 = local read "SEM Scan Parameters"() -> (w3482:T26)
            n4318 = Unbundle By Name(w3482) -> ("WD (mm)"=w3484:sgl[][], "X tiles"=w3480:u8, "Y tiles"=w3479:u8)
            n4319 = call "2D array edit.vi"("Data Entry Limits:Increment"=0.001, "Display Format:Precision"=u8 4, "Rows"=w3479, "Columns"=w3480, "Caption.Text"="WD (mm)", "Input array"=w3484) -> ("Output array"=w3478:sgl[][])  [unwired: 5 in]
            n4320 = Array Size(array=w3478) -> (size(s)=w3477:i32[])
            n4321 = Index Array(array=w3477) -> (element #1=w3476:i32, element #2=w3475:i32)  [unwired: 2 in]
            n4322 = Bundle By Name(cluster=w3482, "WD (mm)"=w3478, "X tiles"=w3475, "Y tiles"=w3476) -> (w3481:T26)
            n4323 = local write "SEM Scan Parameters"(w3481) -> ()
          }
          event "SEM Scan Parameters.X stig": Mouse Down; "SEM Scan Parameters.X stig": Value Change {
            n4324 = event-data() -> ()  [unwired: 5 out]
            n4325 = local read "SEM Scan Parameters"() -> (w3494:T26)
            n4326 = Unbundle By Name(w3494) -> ("X stig"=w3496:sgl[][], "X tiles"=w3492:u8, "Y tiles"=w3491:u8)
            n4327 = call "2D array edit.vi"("Data Entry Limits:Increment"=0.1, "Display Format:Precision"=u8 2, "Rows"=w3491, "Columns"=w3492, "Caption.Text"="X stig (%)", "Input array"=w3496) -> ("Output array"=w3489:sgl[][])  [unwired: 5 in]
            n4328 = Array Size(array=w3489) -> (size(s)=w3490:i32[])
            n4329 = Index Array(array=w3490) -> (element #1=w3488:i32, element #2=w3487:i32)  [unwired: 2 in]
            n4330 = Bundle By Name(cluster=w3494, "X stig"=w3489, "X tiles"=w3487, "Y tiles"=w3488) -> (w3493:T26)
            n4331 = local write "SEM Scan Parameters"(w3493) -> ()
          }
          event "SEM Scan Parameters.Y stig": Mouse Down; "SEM Scan Parameters.Y stig": Value Change {
            n4332 = event-data() -> ()  [unwired: 5 out]
            n4333 = local read "SEM Scan Parameters"() -> (w3506:T26)
            n4334 = Unbundle By Name(w3506) -> ("Y stig"=w3508:sgl[][], "X tiles"=w3504:u8, "Y tiles"=w3503:u8)
            n4335 = call "2D array edit.vi"("Data Entry Limits:Increment"=0.1, "Display Format:Precision"=u8 2, "Rows"=w3503, "Columns"=w3504, "Caption.Text"="Y stig (%)", "Input array"=w3508) -> ("Output array"=w3501:sgl[][])  [unwired: 5 in]
            n4336 = Array Size(array=w3501) -> (size(s)=w3502:i32[])
